vi "Secondary Flow.vi"(0 "NDHX Heat Transfer (W)":dbl, 1 "Dctl (m)":dbl, 2 "Sec Cold Temp (K)":dbl, 3 "MHX Tube Diameter (m)":dbl, 4 "Sec Loop Width (m)":dbl, 5 "MHX Tube Pitch (m)":dbl, 6 "Sec Hot Temp (K)":dbl, 7 "MHX Heat Transfer (W)":dbl, 9 "Pipe Diameter (m)":dbl, 10 "NDHX Number of Tubes":dbl, 11 "Sec Mass Flow (kg/s)":dbl, 12 "Sec Loop Height (m)":dbl, 13 "Pipe XArea (m^2)":dbl, 14 "Sec Delta T (K)":dbl, 15 "MHX Length (m)":dbl, 16 "Time":dbl, 17 "NDHX Tube Diameter (m)":dbl, 18 "Sec Ave Temp (K)":dbl, 19 "Number of MHX Baffles":dbl, 27 "NDHX Tube Length (m)":dbl) -> (20 "Secondary Cold Temperature (K)":dbl, 21 "Sec Mass Flow (kg/s)":dbl, 22 "Cp of FLiNaK (J/kgK)":dbl, 23 "FLiNaK Ave Viscosity (Pa-s)":dbl, 24 "Sec Hot Temp (K)":dbl)   [LabVIEW 2019]
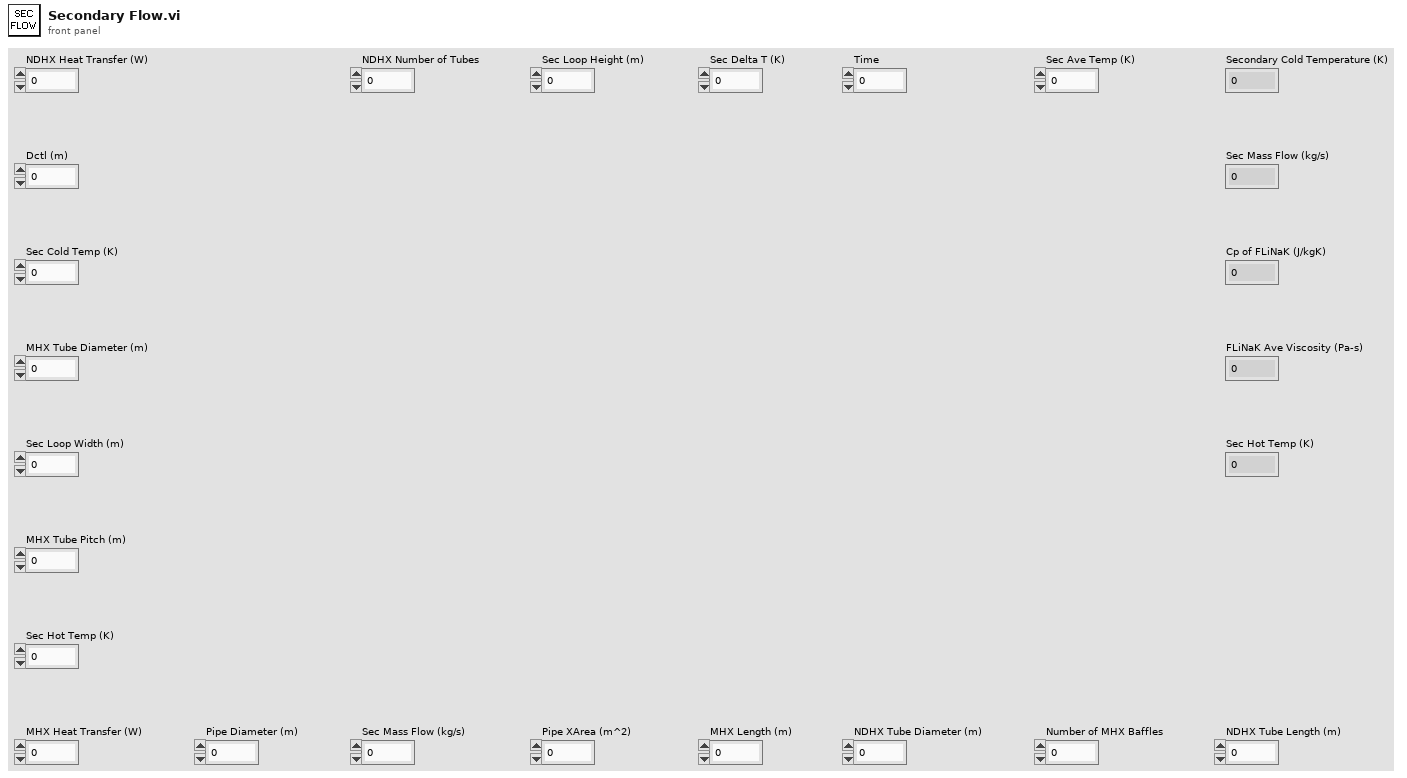
[diagram p1: front panel]
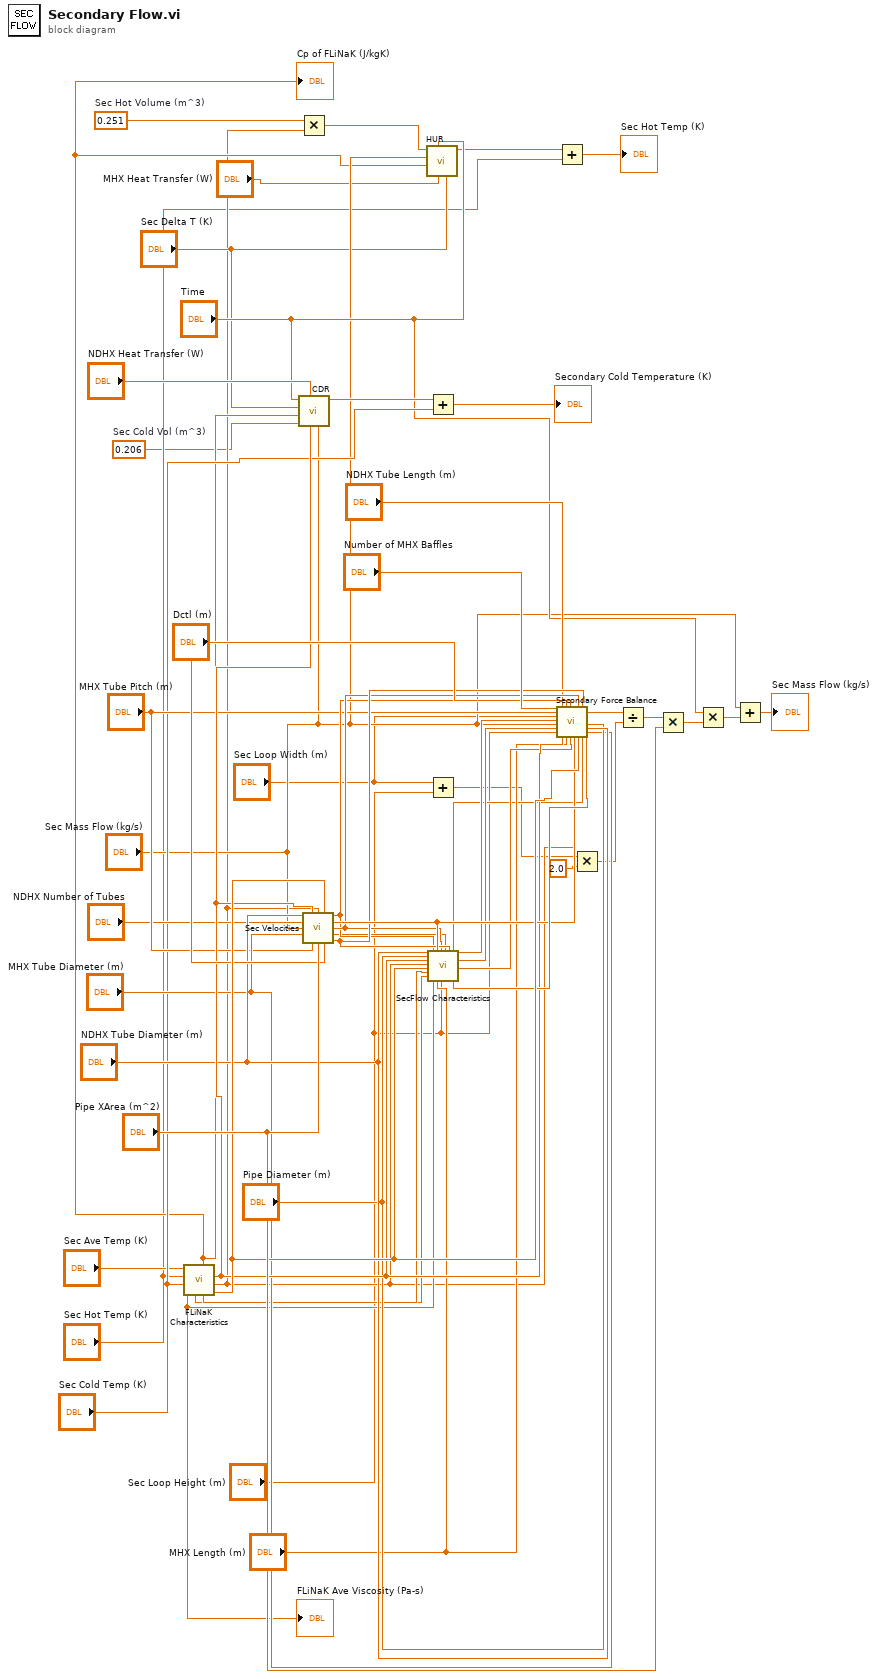
[diagram p0: block diagram]
diagram:
  w1 = 0.206  # Sec Cold Vol (m^3)
  w8 = 0.251  # Sec Hot Volume (m^3)
  n1 = call "FLiNaK Characteristics.vi"("Sec Cold Temp (K)"="Sec Cold Temp (K)", "Sec Hot Temp (K)"="Sec Hot Temp (K)", "Sec Ave Temp (K)"="Sec Ave Temp (K)") -> ("Sec Ave Density (kg/m^3) 3"=w46:dbl, "Sec Hot Density (kg/m^3) 2"=w10:dbl, "Sec Cold Density (kg/m^3)"=w41:dbl, "FLiNaK Cold Viscosity (Pa-s)"=w27:dbl, "Cp of FLiNaK (J/kgK)"=w13:dbl, "FLiNaK Hot Viscosity (Pa-s)"=w26:dbl, "FLiNaK Ave Viscosity (Pa-s)"=w28:dbl)  [unwired: 2 in]
  "Cp of FLiNaK (J/kgK)" <- w13
  "FLiNaK Ave Viscosity (Pa-s)" <- w28
  n2 = Multiply(x=w8, y=w10) -> (x*y=w9:dbl)
  n3 = call "CDR.vi"("Mass Flow (kg/s)"="Sec Mass Flow (kg/s)", "Density (kg/m^3)"=w41, "HX Power (W)"="NDHX Heat Transfer (W)", "Cold Vol (m^3)"=w1, "Cp (J/kgK)"=w13, "Delta T (K)"="Sec Delta T (K)", "Time (s)"="Time") -> ("Cooldown (K)"=w18:dbl)  [unwired: 4 in]
  n4 = call "Sec Velocities.vi"("NDHX Tube Diameter (m)"="NDHX Tube Diameter (m)", "Sec Cold Density (kg/m^3)"=w41, "Sec Hot Density (kg/m^3) in"=w10, "Sec Ave Density (kg/m^3) 3"=w46, "NDHX Number of Tubes"="NDHX Number of Tubes", "Sec Mass Flow (kg/s)"="Sec Mass Flow (kg/s)", "MHX Tube Diameter (m)"="MHX Tube Diameter (m)", "MHX Tube Pitch (m)"="MHX Tube Pitch (m)", "Pipe XArea (m^2)"="Pipe XArea (m^2)", "Dctl (m)"="Dctl (m)") -> ("Shell Crossflow Area (m^2)"=w31:dbl, "Sec Cold Velocity (m/s)"=w42:dbl, "Sec Hot Velocity (m/s)"=w39:dbl, "Sec MHX Velocity (m/s)"=w25:dbl, "Sec NDHX Velocity (m/s)"=w40:dbl)  [unwired: 1 in]
  n5 = call "HUR.vi"("Delta T (K)"="Sec Delta T (K)", "Heating Power (W)"="MHX Heat Transfer (W)", "Time"="Time", "Cp (J/kgK)"=w13, "Mass Flow (kg/s)"="Sec Mass Flow (kg/s)", "Hot Mass (kg)"=w9) -> ("HUR (K)"=w3:dbl)  [unwired: 4 in, 1 out]
  n6 = Add(x=w18, y="Sec Cold Temp (K)") -> (x+y=→"Secondary Cold Temperature (K)":dbl)
  n7 = Add(x="Sec Loop Width (m)", y="Sec Loop Height (m)") -> (x+y=w5:dbl)
  n8 = call "SecFlow Characteristics.vi"("NDHX Tube Diameter (m)"="NDHX Tube Diameter (m)", "Pipe Diameter (m)"="Pipe Diameter (m)", "Sec Cold Density (kg/m^3)"=w41, "Sec Hot Density (kg/m^3) in"=w10, "Sec Ave Density (kg/m^3) 3"=w46, "FLiNaK Cold Viscosity (Pa-s)"=w27, "FLiNaK Hot Viscosity (Pa-s)"=w26, "Shell Crossflow Area (m^2)"=w31, "FLiNaK Ave Viscosity (Pa-s)"=w28, "Sec Cold Velocity (m/s)"=w42, "MHX Length (m)"="MHX Length (m)", "Sec Hot Velocity (m/s)"=w39, "Sec Loop Height (m)"="Sec Loop Height (m)", "Sec MHX Velocity (m/s)"=w25, "Sec NDHX Velocity (m/s)"=w40) -> ("Numeric"=w23:dbl, "EA Friction Factor"=w43:dbl, "AB Friction Factor"=w32:dbl, "BC Friction Factor"=w36:dbl, "CEFriction Factor"=w34:dbl)  [unwired: 4 in, 4 out]
  n9 = Add(x=w3, y="Sec Hot Temp (K)") -> (x+y=→"Sec Hot Temp (K)":dbl)
  n10 = call "Secondary Force Balance.vi"("Number of MHX Baffles"="Number of MHX Baffles", "MHX Tube Pitch (m)"="MHX Tube Pitch (m)", "Sec Loop Width (m)"="Sec Loop Width (m)", "AB Friction Factor"=w32, "Sec Mass Flow (kg/s)"="Sec Mass Flow (kg/s)", "BC Friction Factor"=w36, "Sec Loop Height (m)"="Sec Loop Height (m)", "NDHX Tube Length (m)"="NDHX Tube Length (m)", "Sec Cold Density (kg/m^3)"=w41, "Dctl (m)"="Dctl (m)", "MHX Length (m)"="MHX Length (m)", "Shell Crossflow Area (m^2)"=w31, "CEFriction Factor"=w34, "Sec Cold Velocity (m/s)"=w42, "Sec Hot Density (kg/m^3) in"=w10, "Sec Hot Velocity (m/s)"=w39, "Sec Ave Density (kg/m^3) 3"=w46, "Sec NDHX Velocity (m/s)"=w40, "Numeric in"=w23, "Pipe Diameter (m)"="Pipe Diameter (m)", "NDHX Tube Diameter (m)"="NDHX Tube Diameter (m)", "MHX Tube Diameter (m)"="MHX Tube Diameter (m)", "EA Friction Factor"=w43) -> ("Force Balance (Pa)"=w50:dbl)  [unwired: 4 in]
  n11 = Multiply(x=w5, y=2.0) -> (x*y=w16:dbl)
  n12 = Divide(x=w50, y=w16) -> (x/y=w51:dbl)
  n13 = Multiply(x=w51, y="Pipe XArea (m^2)") -> (x*y=w47:dbl)
  n14 = Multiply(x="Time", y=w47) -> (x*y=w48:dbl)
  n15 = Add(x="Sec Mass Flow (kg/s)", y=w48) -> (x+y=→"Sec Mass Flow (kg/s)":dbl)
